vi "Set Acquisition Configuration.vi"(8 "error in (no error)":errorcluster, 11 "CCDCamera in":refnum<class "CCDCamera.lvclass">) -> (0 "error out":errorcluster, 3 "CCDCamera out":refnum<class "CCDCamera.lvclass">)   [LabVIEW 2018, in "CCDCamera.lvclass"]
doc: "Set the camera configuration\n\nThis function records the given operating parameters in the camera. However, the parameters will only bewritten if their last value is different from the most recent one."
uses:
  CCDCamera.lvclass
panel:
  out "x != y? 2":T1
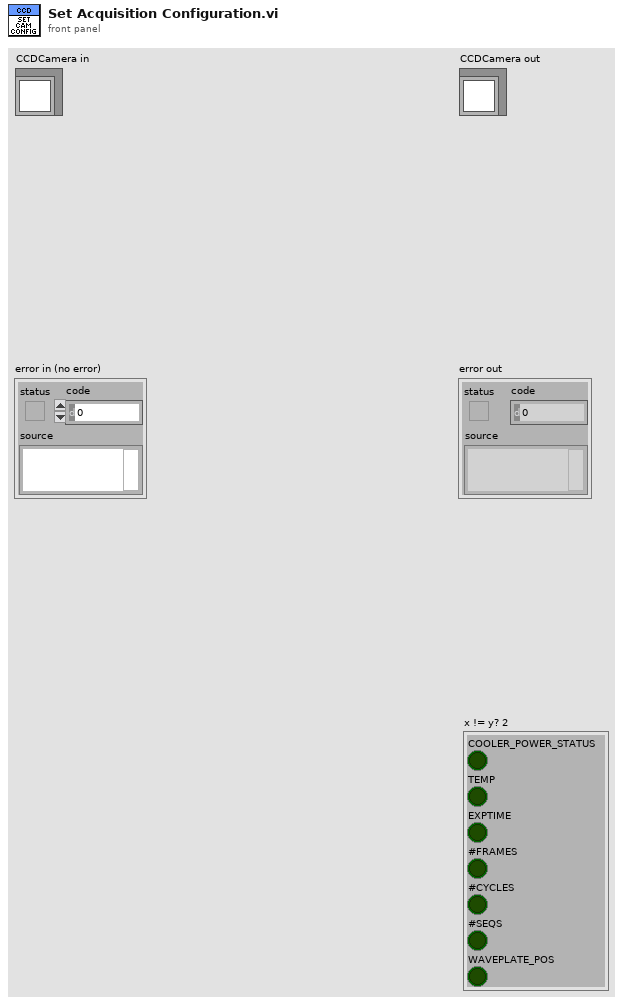
[diagram p1: front panel]
types:
  T1 = cluster{"COOLER_POWER_STATUS":bool, "TEMP":bool, "EXPTIME":bool, "#FRAMES":bool, "#CYCLES":bool, "#SEQS":bool, "WAVEPLATE_POS":bool}
  T2 = cluster{"COOLER_POWER_STATUS":u16, "TEMP":i32, "EXPTIME":dbl, "#FRAMES":u32, "#CYCLES":u32, "#SEQS":u32, "WAVEPLATE_POS":u16}
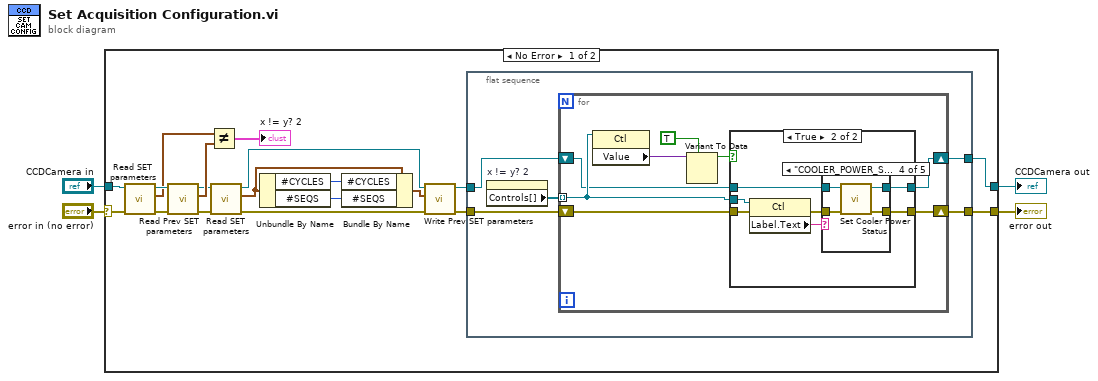
[diagram p0: block diagram]
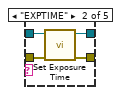
[diagram p4: hidden frame]
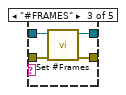
[diagram p5: hidden frame]
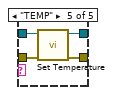
[diagram p6: hidden frame]
diagram:
  n1 = case shown="No Error" "error in (no error)" {
    selector: "error in (no error)" -> [w5 w65]
    tunnel: [w23 w65] -> w4
    tunnel: [w22 w64] -> w3
    tunnel: "CCDCamera in" -> [w6 w64]
    frame No Error {
      n2 = call-dynamic "Read SET parameters.vi"("error in (no error)"=w5, "Simulated_CCD_Camera in"=w6) -> ("error out"=w21:errorcluster, "New SET parameters"=w18:T2, "Simulated_CCD_Camera out"=w20:refnum<class "CCDCamera.lvclass">)  [unwired: 7 in]
      n3 = call-dynamic "Read Prev SET parameters.vi"("error in (no error)"=w21, "Simulated_CCD_Camera in"=w20) -> ("error out"=w13:errorcluster, "Prev SET parameters"=w19:T2, "Simulated_CCD_Camera out"=w14:refnum<class "CCDCamera.lvclass">)  [unwired: 7 in]
      n4 = Not Equal?(x=w18, y=w19) -> (x != y?=→"x != y? 2":T1)
      n5 = call-dynamic "Read SET parameters.vi"("error in (no error)"=w13, "Simulated_CCD_Camera in"=w14) -> ("error out"=w10:errorcluster, "New SET parameters"=w16:T2, "Simulated_CCD_Camera out"=w17:refnum<class "CCDCamera.lvclass">)  [unwired: 7 in]
      n6 = Unbundle By Name(w16) -> ("#CYCLES"=w9:u32, "#SEQS"=w8:u32)
      n7 = Bundle By Name(cluster=w16, "#CYCLES"=w9, "#SEQS"=w8) -> (w15:T2)
      n8 = call-dynamic "Write Prev SET parameters.vi"("error in (no error)"=w10, "Prev SET parameters"=w15, "Simulated_CCD_Camera in"=w17) -> ("error out"=w11:errorcluster, "Simulated_CCD_Camera out"=w12:refnum<class "CCDCamera.lvclass">)  [unwired: 7 in]
      n9 = flat-sequence {
        tunnel: w11 -> [w24]
        tunnel: [w28] -> w23
        tunnel: w12 -> [w27]
        tunnel: [w26] -> w22
        frame #0 {
          n10 = property on="x != y? 2" class="Clust (strict)"() -> ("Controls[]"=w25:refnum<vi>[])  [unwired: 2 in, 2 out]
          n11 = for {
            tunnel: w25 -> [w35] mode=indexing
            shift-right: [w29] -> w28
            shift-left: w24 -> [w36]
            shift-right: [w30] -> w26
            shift-left: w27 -> [w31]
            n12 = property class="Ctl"(reference=w35) -> ("Value"=w34:variant)  [unwired: 1 in, 2 out]
            n13 = Variant To Data(type=TRUE, Variant=w34) -> (data=w32:bool)  [unwired: 1 in, 1 out]
            n14 = case shown="True" w32 {
              tunnel: w35 -> [_ w45]
              tunnel: [w38 w39] -> w29
              tunnel: w36 -> [w38 w43]
              tunnel: w31 -> [w37 w42]
              tunnel: [w37 w41] -> w30
              frame False {
              }
              frame True {
                n15 = property class="Ctl"(reference=w45, error in=w43) -> (error out=w40:errorcluster, "Label.Text"=w44:string)  [unwired: 1 out]
                n16 = case shown="\"COOLER_POWER_STATUS\"" w44 {
                  tunnel: w42 -> [w47 w51 w54 w58 w63]
                  tunnel: [w47 w50 w55 w59 w62] -> w41
                  tunnel: w40 -> [w46 w49 w53 w57 w61]
                  tunnel: [w46 w48 w52 w56 w60] -> w39
                  frame "False", Default {
                  }
                  frame "EXPTIME" {
                    n17 = call-dynamic "Set Exposure Time.vi"("error in (no error)"=w49, "CCDCamera in"=w51) -> ("error out"=w48:errorcluster, "CCDCamera out"=w50:refnum<class "CCDCamera.lvclass">)  [unwired: 8 in]
                  }
                  frame "#FRAMES" {
                    n18 = call-dynamic "Set #Frames.vi"("error in (no error)"=w53, "CCDCamera in"=w54) -> ("error out"=w52:errorcluster, "CCDCamera out"=w55:refnum<class "CCDCamera.lvclass">)  [unwired: 8 in]
                  }
                  frame "COOLER_POWER_STATUS" {
                    n19 = call-dynamic "Set Cooler Power Status.vi"("error in (no error)"=w57, "CCDCamera in"=w58) -> ("error out"=w56:errorcluster, "CCDCamera out"=w59:refnum<class "CCDCamera.lvclass">)  [unwired: 8 in]
                  }
                  frame "TEMP" {
                    n20 = call-dynamic "Set Temperature.vi"("error in (no error)"=w61, "CCDCamera in"=w63) -> ("error out"=w60:errorcluster, "CCDCamera out"=w62:refnum<class "CCDCamera.lvclass">)  [unwired: 8 in]
                  }
                }
              }
            }
          }
        }
      }
    }
    frame Error {
    }
  }
  "error out" <- w4
  "CCDCamera out" <- w3
